vi "Calculate moves.vi"(7 "Position":refnum<class "Position.lvclass">, 8 "error in (no error)":errorcluster, 10 "Source":T1={"File"=enum."d", "Rank"=enum."4"}, 11 "King in":refnum<class "King.lvclass">) -> (0 "error out":errorcluster, 2 "Moves":refnum<class "Move.lvclass">[](array[class]), 3 "King out":refnum<class "King.lvclass">)   [LabVIEW 2016, in "Chesslib.lvlib" / "King.lvclass"]
uses:
  King.lvclass
  Moves/Move/Move.lvclass
  typedef/Square.ctl
  typedef/File.ctl
  typedef/Rank.ctl
  Position/Position.lvclass
  Moves/CastleRestricting/CastleRestricting.lvclass
  C:/Users/GRTaggJ/Documents/Projects/chesslib/Moves/Move/Move.lvclass
  Chesslib.lvlib
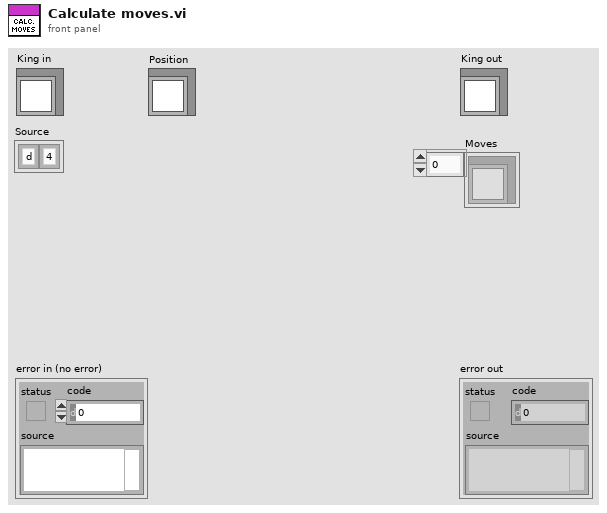
[diagram p1: front panel]
types:
  T1 = typedef "Chesslib.lvlib/Square.ctl" = cluster{"File":T2, "Rank":T3}
  T2 = typedef "Chesslib.lvlib/File.ctl" = enum8{"a", "b", "c", "d", "e", "f", "g", "h"}
  T3 = typedef "Chesslib.lvlib/Rank.ctl" = enum8{"1", "2", "3", "4", "5", "6", "7", "8"}
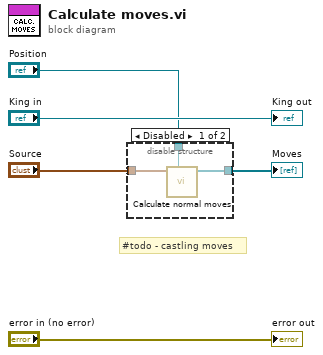
[diagram p0: block diagram]
diagram:
  # "#todo - castling moves"
  n1 = disable-structure shown="Disabled" {
    disable-tunnel: [w8 _] -> w4
    disable-tunnel: "Position" -> [w7 _]
    disable-tunnel: "Source" -> [w6 _]
    frame Disabled {
      n2 = call "Calculate normal moves.vi"("Position in"=w7, "Source"=w6) -> ("Normal moves"=w8:refnum<class "CastleRestricting.lvclass">[])  [unwired: 9 in]
    }
    frame Enabled {
    }
  }
  "Moves" <- w4
  "error out" <- "error in (no error)"
  "King out" <- "King in"
